vi "_New Group.vi"(8 "error in (no error)":errorcluster, 10 "Group Config":refnum<class "Group Config.lvclass">, 11 "Loop Data in":T1) -> (0 "error out":errorcluster, 2 "Group":refnum<class "Group.lvclass">, 3 "Loop Data":T1)   [LabVIEW 2020, in "Vecto.lvlib" / "ChannelService.lvclass"]
uses:
  ChannelService.lvclass
  Group Config/Group Config.lvclass
  Channel Config/Channel Config.lvclass
  Group/Group.lvclass
  Loop Data.ctl
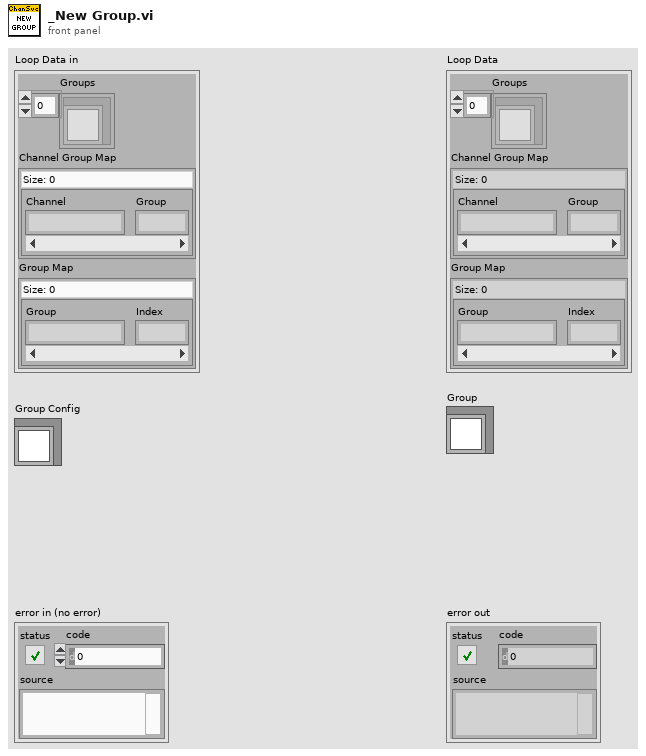
[diagram p1: front panel]
types:
  T1 = typedef "Vecto.lvlib/ChannelService.lvclass/Loop Data.ctl" = cluster{"Groups":refnum<class "Group.lvclass">[], "Channel Group Map":map{string, i32}, "Group Map":map{string, i32}}
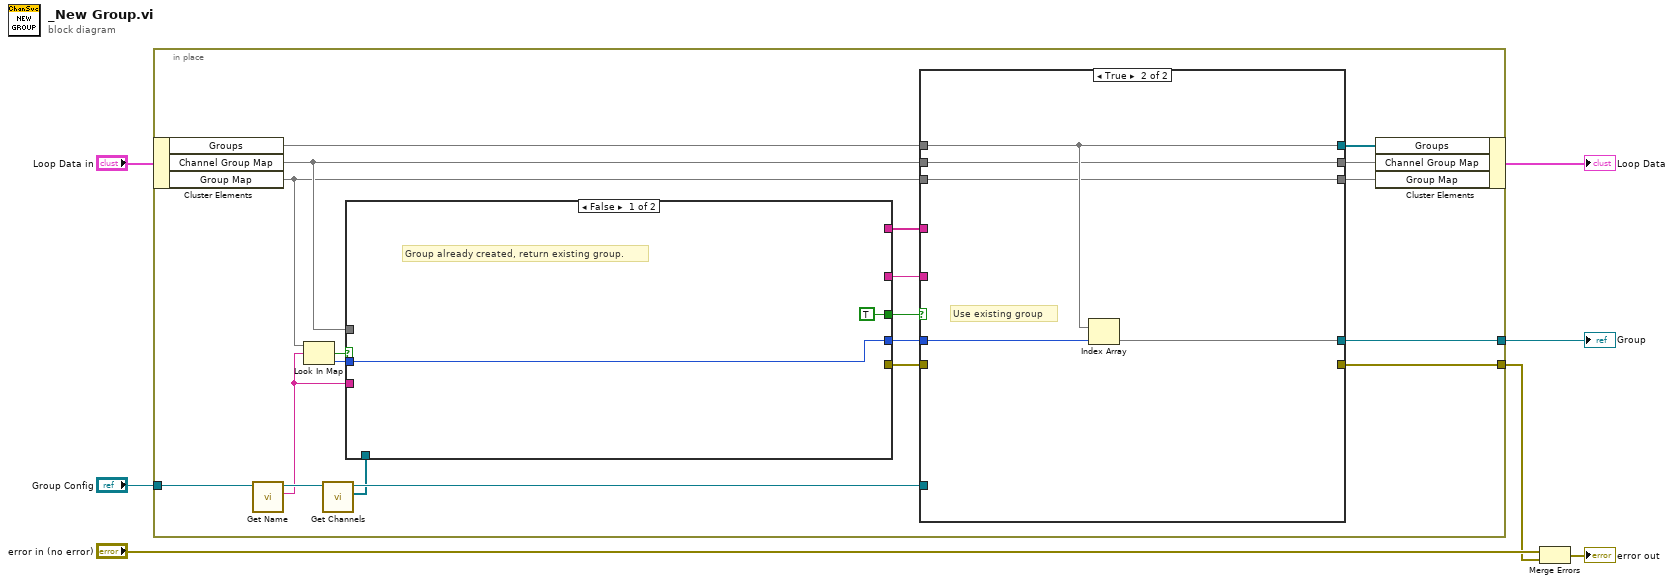
[diagram p0: block diagram]
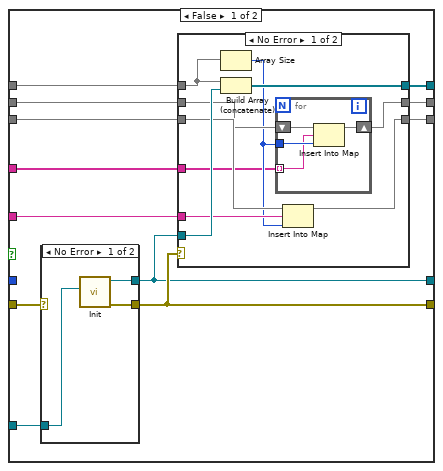
[diagram p2: hidden frame]
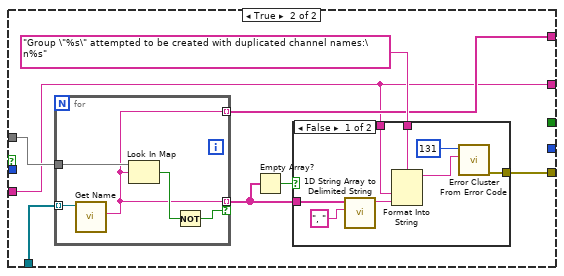
[diagram p5: hidden frame]
diagram:
  n1 = in-place {
    in-place-border: "Group Config" -> [w25]
    in-place-border: [w24] -> w4
    in-place-border: [w15] -> w2
    n2 = in-place-cluster #1("Loop Data in") -> ("Groups"=w23, "Channel Group Map"=w21, "Group Map"=w18)
    n3 = call "Get Name.vi"("Group Config in"=w25) -> ("Name"=w13:string, "Group Config out"=w14:refnum<class "Group Config.lvclass">)  [unwired: 8 in, 1 out]
    n4 = Look In Map(map=w18, key=w13) -> (key not found?=w27:bool, value=w10:i32)  [unwired: 1 in]
    n5 = call "Get Channels.vi"("Group Config in"=w14) -> ("Channels"=w11:refnum<class "Channel Config.lvclass">[], "Group Config out"=w12:refnum<class "Group Config.lvclass">)  [unwired: 8 in, 1 out]
    n6 = case shown="False" w27 {
      tunnel: w13 -> [_ w71]
      tunnel: w21 -> [_ w75]
      tunnel: [_ w74] -> w26
      tunnel: [_ w72] -> w17
      tunnel: [_ w71] -> w16
      tunnel: w11 -> [_ w70]
      tunnel: w10 -> [w66 _]
      tunnel: [TRUE _] -> w9
      tunnel: [w66 _] -> w8
      frame False {
        # "Group already created, return existing group."
      }
      frame True {
        n7 = for {
          tunnel: w75 -> [w88]
          tunnel: w70 -> [w85] mode=indexing
          tunnel: [w84] -> w69 mode=indexing if=w86
          tunnel: [w84] -> w72 mode=indexing
          n8 = call "Get Name.vi"("Channel Config in"=w85) -> ("Name"=w84:string)  [unwired: 8 in, 2 out]
          n9 = Look In Map(map=w88, key=w84) -> (key not found?=w87:bool)  [unwired: 1 in, 1 out]
          n10 = Not(x=w87) -> (.not. x?=w86:bool)
        }
        n11 = Empty Array?(array=w69) -> (empty?=w68:bool)
        n12 = case shown="False" w68 {
          tunnel: [w83 _] -> w74
          tunnel: "Group \"%s\" attempted to be created with duplicated channel names:\n%s" ("format string") -> [w80 _]
          tunnel: w71 -> [w77 _]
          tunnel: w69 -> [w76 _]
          frame False {
            n13 = call <vilib>:"1D String Array to Delimited String.vi"("delimiter"=", ", "string array"=w76) -> ("delimited string"=w79:string)  [unwired: 9 in]
            n14 = Format Into String(format string=w80, w77, w79) -> (resulting string=w78:string)  [unwired: 2 in, 1 out]
            n15 = call <vilib>:"Error Cluster From Error Code.vi"("error message (\"\")"=w78, "error code (0)"=131) -> ("error out"=w83:errorcluster)  [unwired: 7 in]
          }
          frame True {
          }
        }
      }
    }
    n16 = case shown="True" w9 {
      tunnel: w26 -> [w39 _]
      tunnel: [w38 _] -> w24
      tunnel: w23 -> [w37 w64]
      tunnel: [w36 w64] -> w22
      tunnel: w21 -> [w35 w63]
      tunnel: [w34 w63] -> w20
      tunnel: [w33 w62] -> w19
      tunnel: w18 -> [w32 w62]
      tunnel: w17 -> [w31 _]
      tunnel: w16 -> [w30 _]
      tunnel: [w29 w65] -> w15
      tunnel: w12 -> [w28 _]
      tunnel: w8 -> [_ w61]
      frame False {
        n17 = case shown="No Error" w39 {
          selector: w39 -> [_ w60]
          tunnel: w28 -> [w57 _]
          tunnel: [w59 w60] -> w38
          tunnel: [w58 _] -> w29
          frame No Error {
            n18 = call "Init.vi"("Group Config"=w57) -> ("error out"=w59:errorcluster, "Group"=w58:refnum<class "Group.lvclass">)  [unwired: 9 in]
          }
          frame Error {
          }
        }
        n19 = case shown="No Error" w38 {
          tunnel: w29 -> [w48 _]
          tunnel: w37 -> [w49 w56]
          tunnel: [w47 w56] -> w36
          tunnel: w35 -> [w43 w55]
          tunnel: [w40 w55] -> w34
          tunnel: [w44 w54] -> w33
          tunnel: w32 -> [w46 w54]
          tunnel: w31 -> [w41 _]
          tunnel: w30 -> [w45 _]
          frame No Error {
            n20 = Array Size(array=w49) -> (size(s)=w42:i32)
            n21 = Build Array (concatenate)(w49, w48) -> (w47:refnum<class "Group.lvclass">[])
            n22 = for {
              shift-right: [w50] -> w40
              shift-left: w43 -> [w53]
              tunnel: w42 -> [w52]
              tunnel: w41 -> [w51] mode=indexing
              n23 = Insert Into Map(map in=w53, key=w51, value=w52) -> (map out=w50:map{string, i32})  [unwired: 2 out]
            }
            n24 = Insert Into Map(map in=w46, key=w45, value=w42) -> (map out=w44:map{string, i32})  [unwired: 2 out]
          }
          frame Error {
          }
        }
      }
      frame True {
        # "Use existing group"
        n25 = Index Array(array=w64, index=w61) -> (element=w65)
      }
    }
    n26 = in-place-cluster #1("Groups"=w22, "Channel Group Map"=w20, "Group Map"=w19) -> (→"Loop Data":cluster{})
  }
  "Group" <- w2
  n27 = Merge Errors("error in (no error)", w4) -> (→"error out":errorcluster)
